vi "GenerateHtmlDoc.vi"() -> ()   [LabVIEW 2024]
panel:
  out "error out":errorcluster
  in  "LvlibPath":path
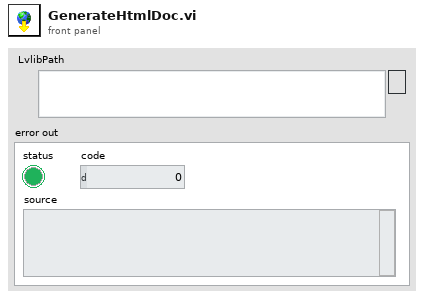
[diagram p1: front panel]
types:
  T1 = enum32{"Custom", "Standard", "Using Panel", "Using SubVI", "Complete"}
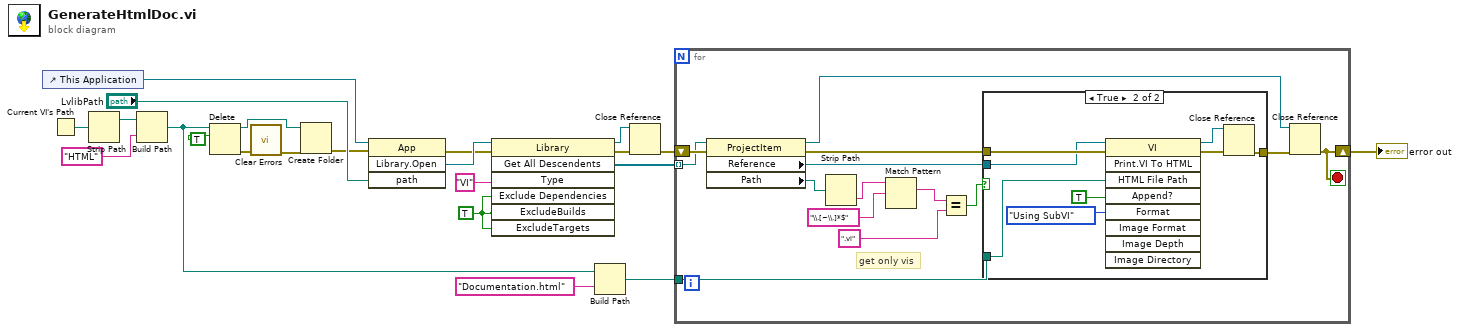
[diagram p0: block diagram]
diagram:
  w16 = TRUE
  n1 = control-ref of="This Application"() -> (w22:refnum<vi>)
  n2 = Current VI's Path() -> (path=w13:path)
  n3 = Strip Path(path=w13) -> (stripped path=w12:path)  [unwired: 1 out]
  n4 = Build Path(base path=w12, name or relative path="HTML") -> (appended path=w8:path)
  n5 = Delete(path (use dialog)=w8, entire hierarchy (F)=TRUE) -> (deleted path=w4:path, error out=w5:errorcluster)  [unwired: 3 in, 1 out]
  n6 = call <vilib>:"Clear Errors.vi"("error in (no error)"=w5) -> ("error out"=w3:errorcluster)  [unwired: 5 in, 1 out]
  n7 = Create Folder(path (use dialog)=w4, error in=w3) -> (error out=w1:errorcluster)  [unwired: 1 in, 2 out]
  n8 = invoke class="App" method="Library.Open"(reference=w22, error in=w1, "path"="LvlibPath") -> (error out=w18:errorcluster, "Open Library"=w21:refnum<vi>)  [unwired: 1 in, 2 out]
  n9 = invoke class="Library" method="Get All Descendents"(reference=w21, error in=w18, "Type"="VI", "Exclude Dependencies"=w16, "ExcludeBuilds"=w16, "ExcludeTargets"=w16) -> (reference out=w19:refnum<vi>, error out=w20:errorcluster, "All Descendents"=w15:refnum<vi>[])  [unwired: 1 in, 4 out]
  n10 = Build Path(base path=w8, name or relative path="Documentation.html") -> (appended path=w2:path)
  n11 = Close Reference(reference=w19, error in (no error)=w20) -> (error out=w9:errorcluster)
  n12 = for {
    tunnel: w15 -> [w35] mode=indexing
    shift-right: [w29] -> w14
    shift-left: w9 -> [w36]
    tunnel: w2 -> [w30]
    stop <- w29 stop-if-true
    # "get only vis"
    n13 = property class="ProjectItem"(reference=w35, error in=w36) -> (reference out=w31:refnum<vi>, error out=w34:errorcluster, "Reference"=w33:refnum<vi>, "Path"=w28:path)
    n14 = Strip Path(path=w28) -> (name=w27:string)  [unwired: 1 out]
    n15 = Match Pattern(string=w27, regular expression="\\.[~\\.]*$") -> (match substring=w23:string)  [unwired: 4 out]
    n16 = Equal?(x=w23, y=".vi") -> (x = y?=w25:bool)
    n17 = case shown="True" w25 {
      tunnel: w34 -> [w37 w45]
      tunnel: w33 -> [_ w44]
      tunnel: [w37 w42] -> w32
      tunnel: w30 -> [_ w40]
      frame False {
        # "no vi"
      }
      frame True {
        n18 = invoke class="VI" method="Print.VI To HTML"(reference=w44, error in=w45, "HTML File Path"=w40, "Append?"=TRUE, "Format"=T1."Using SubVI") -> (reference out=w41:refnum<vi>, error out=w43:errorcluster)  [unwired: 4 in, 7 out]
        n19 = Close Reference(reference=w41, error in (no error)=w43) -> (error out=w42:errorcluster)
      }
    }
    n20 = Close Reference(reference=w31, error in (no error)=w32) -> (error out=w29:errorcluster)
  }
  "error out" <- w14
